vi "solar_type Get Items (Variants).vi"(4 "Include Cluster Prefix? (F)":bool, 6 "Prefix":string, 8 "error in (no error)":errorcluster, 11 "Variant":variant) -> (0 "error out":errorcluster, 1 "Variant Name":string, 2 "Variant Type":T1, 3 "Items":T2[](array[typedef]))   [LabVIEW 2018]
doc: "This returns the data type, name and variant data of each item in the variant."
uses:
  solar_type Item Type.ctl
  solar_type Item.ctl
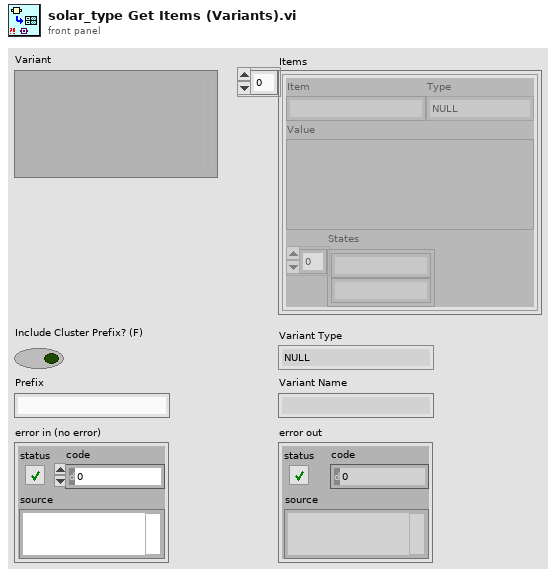
[diagram p1: front panel]
types:
  T1 = typedef "solar_type Item Type.ctl" = enum16{"NULL", "UNKNOWN", "CLUSTER", "I8", "I16", "I32", "I64", "U8", "U16", "U32", "U64", "U8_ENUM", "U16_ENUM", "U32_ENUM", "SGL", "DBL", "BOOLEAN", "STRING", "PATH", "VISA", "TAG", "TIME", "I8_1D", "I16_1D", "I32_1D", "I64_1D", "U8_1D", "U16_1D", "U32_1D", "U64_1D", "U8_ENUM_1D", "U16_ENUM_1D", "U32_ENUM_1D", "SGL_1D", "DBL_1D", "BOOLEAN_1D", "STRING_1D", "PATH_1D", "VISA_1D", "TAG_1D", "TIME_1D", "I8_2D", "I16_2D", "I32_2D", "I64_2D", "U8_2D", "U16_2D", "U32_2D", "U64_2D", "U8_ENUM_2D", "U16_ENUM_2D", "U32_ENUM_2D", "SGL_2D", "DBL_2D", "BOOLEAN_2D", "STRING_2D", "PATH_2D", "VISA_2D", "TAG_2D", "TIME_2D"}
  T2 = typedef "solar_type Item.ctl" = cluster{"Item":string, "Type":T1, "Value":variant, "States":string[]}
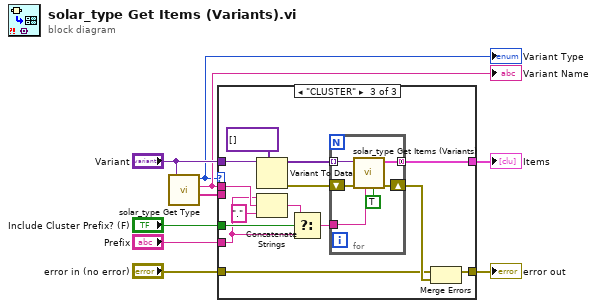
[diagram p0: block diagram]
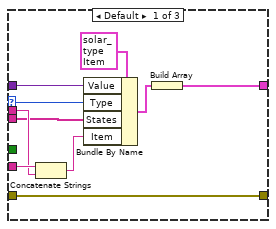
[diagram p2: hidden frame]
diagram:
  n1 = call "solar_type Get Type.vi"("Variant"="Variant") -> ("Type"=w4:T1, "Name"=w5:string, "Enum Names"=w9:string[])  [unwired: 4 in]
  "Variant Name" <- w5
  "Variant Type" <- w4
  n2 = case shown="\"CLUSTER\"" w4 {
    selector: w4 -> [w14 _ _]
    tunnel: "Variant" -> [w12 _ w34]
    tunnel: w5 -> [w18 _ w30]
    tunnel: "Include Cluster Prefix? (F)" -> [_ _ w31]
    tunnel: "Prefix" -> [w19 _ w26]
    tunnel: [w15 _ w25] -> w3
    tunnel: w9 -> [w11 _ _]
    tunnel: "error in (no error)" -> [w10 w20 w22]
    tunnel: [w10 w20 w21] -> w1
    frame Default {
      n3 = Concatenate Strings(w19, w18) -> (w13:string)
      n4 = Bundle By Name(cluster=T2 {"Item"="", "Type"=enum."NULL", "Value"=variant, "States"=[]} ("Item"), "Value"=w12, "Type"=w14, "States"=w11, "Item"=w13) -> (w16:T2)
      n5 = Build Array(w16) -> (w15:T2[])
    }
    frame "NULL" {
      # "Invalid parameter"
    }
    frame "CLUSTER" {
      n6 = Variant To Data(type=variant[] [], Variant=w34) -> (data=w32:variant[], error out=w24:errorcluster)  [unwired: 1 in]
      n7 = Concatenate Strings(w26, w30, "." ("string")) -> (w28:string)
      n8 = Select(t=w28, s=w31, f=w26) -> (s? t:f=w27:string)
      n9 = for {
        tunnel: w32 -> [w40] mode=indexing
        tunnel: w27 -> [w36]
        tunnel: [w37] -> w25 mode=concatenating
        shift-right: [w38] -> w23
        shift-left: w24 -> [w39]
        n10 = call "solar_type Get Items (Variants).vi"("Include Cluster Prefix? (F)"=TRUE, "Prefix"=w36, "error in (no error)"=w39, "Variant"=w40) -> ("error out"=w38:errorcluster, "Items"=w37:T2[])  [unwired: 4 in, 2 out]
      }
      n11 = Merge Errors(w22, w23) -> (w21:errorcluster)
    }
  }
  "Items" <- w3
  "error out" <- w1
